vi "Image Size.vi"   [LabVIEW 2020, in "g_ar_toolkit.image.lvlib"]
uses:
  g_ar_toolkit.image.lvlib
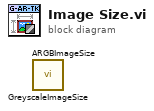
[diagram p0: block diagram]
diagram:
  n1 = call "GreyscaleImageSize.vi"() -> ()  [unwired: 9 in, 3 out]
  n2 = call "ARGBImageSize.vi"() -> ()  [unwired: 9 in, 3 out]
